vi "1a - Local variable.vi"() -> ()   [LabVIEW 2010]
panel:
  in  "stop":bool
  out "Chart 3":i32(graph)
  out "Chart 2":dbl(graph)
  out "Chart 1":dbl(graph)
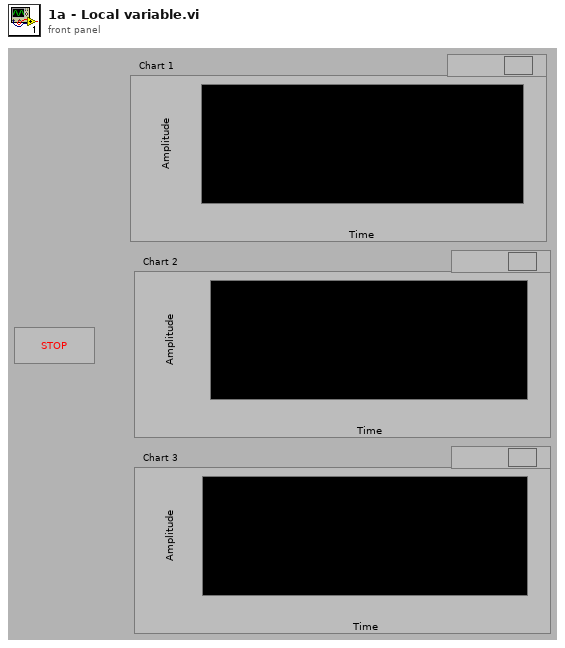
[diagram p1: front panel]
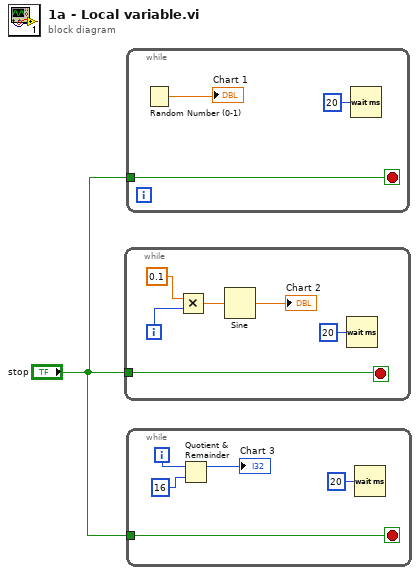
[diagram p0: block diagram]
diagram:
  n1 = while {
    tunnel: "stop" -> [w2]
    i -> [w5]
    stop <- w2 stop-if-true
    n2 = Multiply(x=0.1, y=w5) -> (x*y=w4:dbl)
    n3 = Sine(x=w4) -> (sin(x)=→"Chart 2":dbl)
    n4 = Wait (ms)(milliseconds to wait=u32 20) -> ()  [unwired: 1 out]
  }
  n5 = while {
    tunnel: "stop" -> [w8]
    stop <- w8 stop-if-true
    n6 = Random Number (0-1)() -> (number: 0 to 1=→"Chart 1":dbl)
    n7 = Wait (ms)(milliseconds to wait=u32 20) -> ()  [unwired: 1 out]
  }
  n8 = while {
    tunnel: "stop" -> [w11]
    i -> [w14]
    stop <- w11 stop-if-true
    n9 = Quotient & Remainder(x=w14, y=16) -> (x-y*floor(x/y)=→"Chart 3":i32)  [unwired: 1 out]
    n10 = Wait (ms)(milliseconds to wait=u32 20) -> ()  [unwired: 1 out]
  }
